vi "Setup multiple ramp in awg_positive.vi"(4 "Channel Name (1)":u16(ring)=1 items=["1"=1, "2"=2, "3"=3, "4"=4], 5 "VISA resource name":refnum<visa-resource-name>="GPIB0::1::INSTR", 7 "End time S":dbl=0.000105, 8 "error in (no error)":errorcluster, 9 "Ramp time S":dbl=0.01, 10 "Delay time S":dbl=0.01, 11 "Sampling Frequency (Hz)":u64=10000000) -> (0 "error out":errorcluster)   [LabVIEW 2021]
uses:
  <vilib>/Waveform/DWDTOps.llb/DWDT Boolean Array to Digital.vi
  <instrlib>/Tektronix AWG 5000 7000 Series/Public/Configure/Channel/Assign Output Waveform (From Waveform List).vi
  <instrlib>/Tektronix AWG 5000 7000 Series/Public/Configure/Configure Output Timing (Sampling Frequency).vi
  <instrlib>/Tektronix AWG 5000 7000 Series/Tektronix AWG 5000 7000 Series.lvlib
panel:
  in  "Ramp time S 2":dbl=0.01
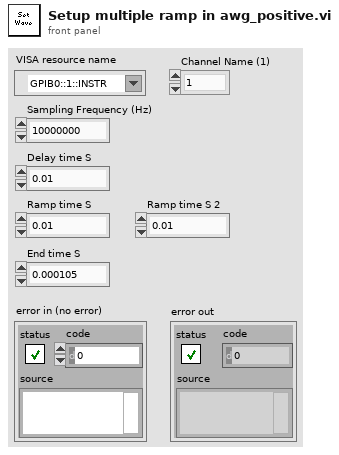
[diagram p1: front panel]
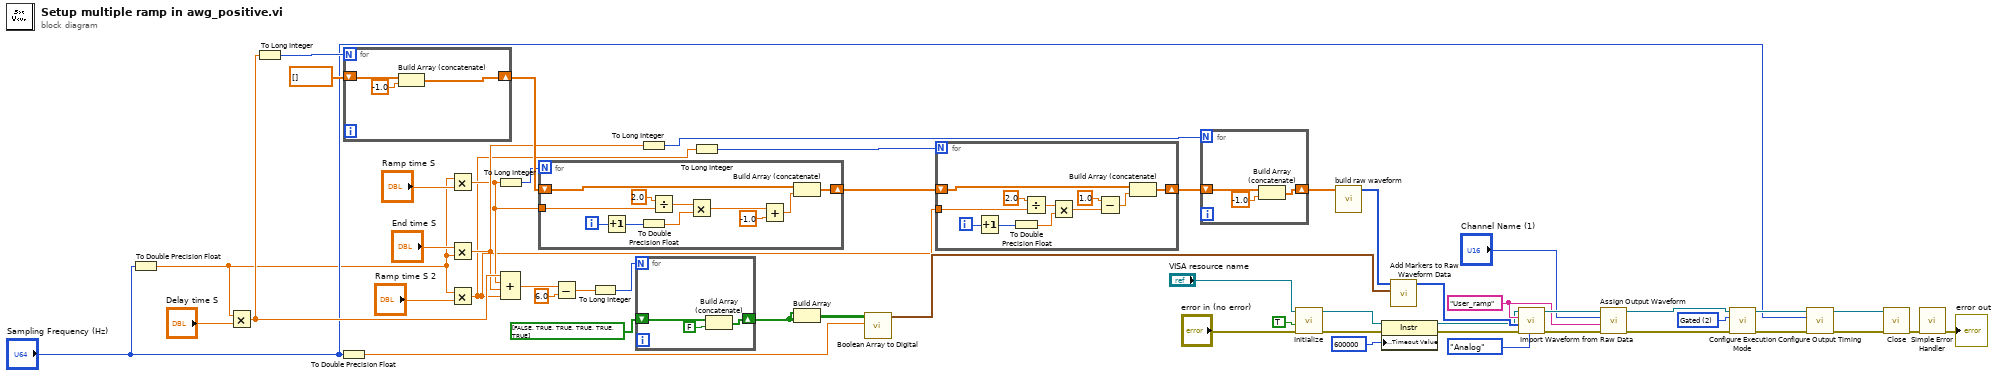
[diagram p0: block diagram]
diagram:
  w24 = u16 2 items=["Continuous", "Triggered", "Gated", "Sequence", "Triggered Continuous"] ("Execution Mode (0 : Continuous)")
  w26 = "User_ramp" ("Waveform Name")
  n1 = To Double Precision Float(number="Sampling Frequency (Hz)") -> (double precision float=w8:dbl)
  n2 = Multiply(x=w8, y="Delay time S") -> (x*y=w34:dbl)
  n3 = To Long Integer(number=w34) -> (32bit integer=w21:i32)
  n4 = To Double Precision Float(number="Sampling Frequency (Hz)") -> (double precision float=w9:dbl)
  n5 = for {
    N: w21 -> [_]
    shift-right: [w54] -> w40
    shift-left: dbl[] [] -> [w55]
    n6 = Build Array (concatenate)(w55, -1.0) -> (w54:dbl[])
  }
  n7 = Multiply(x=w8, y="Ramp time S") -> (x*y=w4:dbl)
  n8 = Multiply(x="End time S", y=w8) -> (x*y=w33:dbl)
  n9 = Multiply(x=w8, y="Ramp time S 2") -> (x*y=w3:dbl)
  n10 = To Long Integer(number=w4) -> (32bit integer=w20:i32)
  n11 = Compound Arithmetic op=ADD(w34, w4, w33, w3) -> (w32:dbl)
  n12 = for {
    N: w20 -> [_]
    shift-right: [w58] -> w6
    shift-left: w40 -> [w60]
    tunnel: w4 -> [w57]
    i -> [w64]
    n13 = Increment(x=w64) -> (x+1=w63:i32)
    n14 = To Double Precision Float(number=w63) -> (double precision float=w56:dbl)
    n15 = Divide(x=2.0, y=w57) -> (x/y=w65:dbl)
    n16 = Multiply(x=w65, y=w56) -> (x*y=w62:dbl)
    n17 = Add(x=w62, y=-1.0) -> (x+y=w59:dbl)
    n18 = Build Array (concatenate)(w60, w59) -> (w58:dbl[])
  }
  n19 = Subtract(x=w32, y=6.0) -> (x-y=w30:dbl)
  n20 = To Long Integer(number=w30) -> (32bit integer=w22:i32)
  n21 = for {
    N: w22 -> [_]
    shift-right: [w67] -> w11
    shift-left: bool[] [FALSE, TRUE, TRUE, TRUE, TRUE, TRUE] -> [w69]
    n22 = Build Array (concatenate)(w69, FALSE) -> (w67:bool[])
  }
  n23 = To Long Integer(number=w33) -> (32bit integer=w1:i32)
  n24 = To Long Integer(number=w3) -> (32bit integer=w2:i32)
  n25 = Build Array(w11, w11) -> (w29:bool[][])
  n26 = call-poly <vilib>:"Boolean Array to Digital.vi"("sample rate"=w9, "boolean array"=w29) -> ("digital waveform"=w18:digitalwaveform)  [unwired: 8 in, 1 out]
  n27 = for {
    N: w2 -> [_]
    shift-right: [w79] -> w5
    shift-left: w6 -> [w80]
    tunnel: w3 -> [w78]
    i -> [w76]
    n28 = Increment(x=w76) -> (x+1=w75:i32)
    n29 = To Double Precision Float(number=w75) -> (double precision float=w73:dbl)
    n30 = Divide(x=2.0, y=w78) -> (x/y=w74:dbl)
    n31 = Multiply(x=w74, y=w73) -> (x*y=w71:dbl)
    n32 = Subtract(x=1.0, y=w71) -> (x-y=w70:dbl)
    n33 = Build Array (concatenate)(w80, w70) -> (w79:dbl[])
  }
  n34 = for {
    N: w1 -> [_]
    shift-right: [w82] -> w36
    shift-left: w5 -> [w83]
    n35 = Build Array (concatenate)(w83, -1.0) -> (w82:dbl[])
  }
  n36 = call <instrlib>:"Initialize.vi"("error in (no error)"="error in (no error)", "Reset (False)"=TRUE ("Reset? (F: No)"), "VISA resource name"="VISA resource name") -> ("error out"=w13:errorcluster, "VISA resource name out"=w15:refnum<visa-resource-name>)  [unwired: 7 in]
  n37 = call "build raw waveform.vi"("Y"=w36) -> ("Raw Waveform Data"=w19:u8[])  [unwired: 10 in]
  n38 = property class="Instr"(reference=w15, error in=w13, "General Settings:Timeout Value"=u32 600000) -> (reference out=w14:refnum<visa-resource-name>, error out=w12:errorcluster)
  n39 = call <instrlib>:"Add Markers to Raw Waveform Data.vi"("Markers"=w18, "Raw Waveform Data"=w19) -> ("Raw Waveform Data with Markers"=w17:u8[])  [unwired: 9 in]
  n40 = call <instrlib>:"Import Waveform from Raw Data.vi"("Representation (1 : Analog)"=enum16{"Integer", "Analog"}."Analog", "error in (no error)"=w12, "Raw Data"=w17, "Waveform Name"=w26, "VISA resource name"=w14) -> ("error out"=w25:errorcluster, "VISA resource name out"=w27:refnum<visa-resource-name>)  [unwired: 5 in]
  n41 = call-poly <instrlib>:"Assign Output Waveform.vi"("error in (no error)"=w25, "Waveform"=w26, "Channel Name (1)"="Channel Name (1)", "VISA resource name"=w27) -> ("error out"=w50:errorcluster, "VISA resource name out"=w51:refnum<visa-resource-name>)  [unwired: 6 in]
  n42 = call <instrlib>:"Configure Execution Mode.vi"("error in (no error)"=w50, "Execution Mode (0 : Continuous)"=w24, "VISA resource name"=w51) -> ("error out"=w48:errorcluster, "VISA resource name out"=w49:refnum<visa-resource-name>)  [unwired: 7 in]
  n43 = call-poly <instrlib>:"Configure Output Timing.vi"("error in (no error)"=w48, "Sampling Frequency (Hz) (100MHz)"="Sampling Frequency (Hz)", "VISA resource name"=w49) -> ("error out"=w46:errorcluster, "VISA resource name out"=w47:refnum<visa-resource-name>)  [unwired: 7 in]
  n44 = call <instrlib>:"Close.vi"("error in (no error)"=w46, "VISA resource name"=w47) -> ("error out"=w45:errorcluster)  [unwired: 9 in]
  n45 = call <vilib>:"Simple Error Handler.vi"("error in (no error)"=w45) -> ("error out"=→"error out":errorcluster)  [unwired: 4 in, 4 out]
